vi "ControlVisibility.vi"(8 "error in (no error)":errorcluster, 9 "Visible":bool, 11 "Controls":refnum<vi>[](array[refnum])) -> (0 "error out":errorcluster)   [LabVIEW 2019]
doc: "Mostra o nasconde gli elementi del front panel"
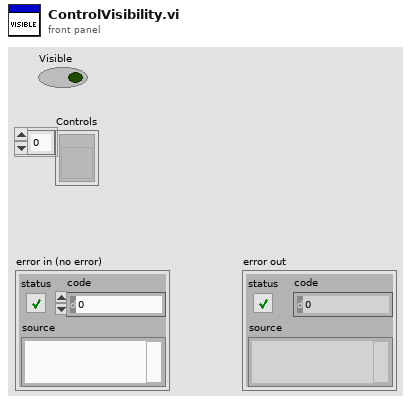
[diagram p1: front panel]
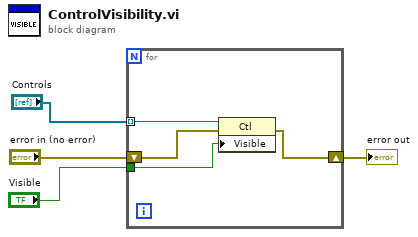
[diagram p0: block diagram]
diagram:
  n1 = for {
    tunnel: "Controls" -> [w8] mode=indexing
    tunnel: "Visible" -> [w7]
    shift-right: [w5] -> w1
    shift-left: "error in (no error)" -> [w6]
    n2 = property class="Ctl"(reference=w8, error in=w6, "Visible"=w7) -> (error out=w5:errorcluster)  [unwired: 1 out]
  }
  "error out" <- w1
